vi "app_star.vi"(5 "TimeStamp [UT]":timestamp format="%<%H:%M:%S%6u\n%Y/%m/%d>T", 6 "error in (no error)":errorcluster, 8 "cat_entry":T1 {"dec" format="%.6g"; "ra" format="%.6g"}, 9 "body (EARTH)":cluster{"type":i8, "number":i8, "name":string}={"type"=0, "number"=3, "name"="EARTH"}) -> (0 "error out":errorcluster, 2 "dec":dbl[unit] format="%_10g", 3 "ra":dbl[unit] format="%_10g")   [LabVIEW 2009]
uses:
  StarAstrometricEntry.ctl
  lib/novas-dll.dll
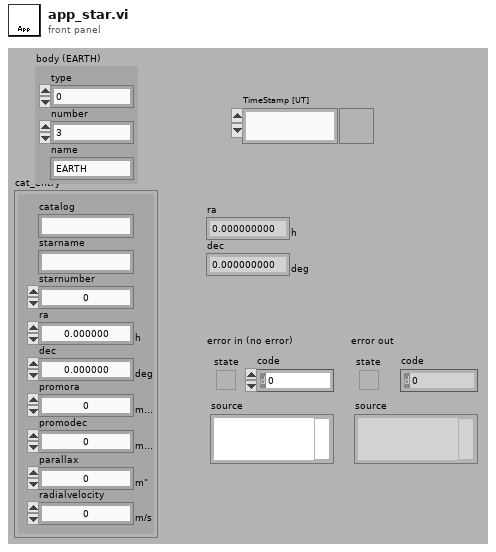
[diagram p1: front panel]
types:
  T1 = typedef "StarAstrometricEntry.ctl" = cluster{"catalog":string, "starname":string, "starnumber":i32, "ra":dbl[unit], "dec":dbl[unit], "promora":dbl[unit], "promodec":dbl[unit], "parallax":dbl[unit], "radialvelocity":dbl[unit]}
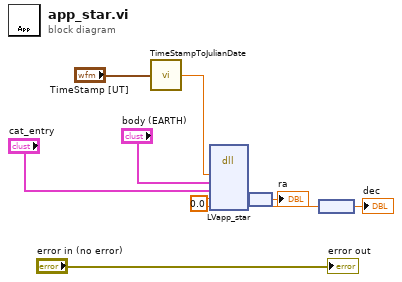
[diagram p0: block diagram]
diagram:
  w9 = 0.0 ("ra")
  n1 = call "TimeStampToJulianDate.vi"("TimeStamp [UT]"="TimeStamp [UT]") -> ("JulianDay"=w2:ext)
  n2 = dll-call lib="C:/Ohana/LV2009/OhanaOS-LV81/Instruments/Novas/lib/novas-dll.dll" fn="LVapp_star"("tjd"=w2, "body (EARTH)"="body (EARTH)", "cat_entry"="cat_entry", "ra"=w9, "dec"=w9) -> ("ra"=w6:dbl, "dec"=w7:dbl)  [unwired: 5 in, 4 out]
  n3 = node(w6) -> (→"ra":dbl[unit])
  n4 = node(w7) -> (→"dec":dbl[unit])
  "error out" <- "error in (no error)"
